vi "Get Ident.vi"(8 "Error In":errorcluster, 11 "reference in":refnum<class "Instrument.lvclass">) -> (0 "Error Out":errorcluster, 2 "Ident":string, 3 "reference out":refnum<class "Instrument.lvclass">)   [LabVIEW 2024, in "HAL.lvlib" / "Instrument.lvclass"]
uses:
  Instrument.lvclass
  Configurations/CFG Base/CFG Base.lvclass
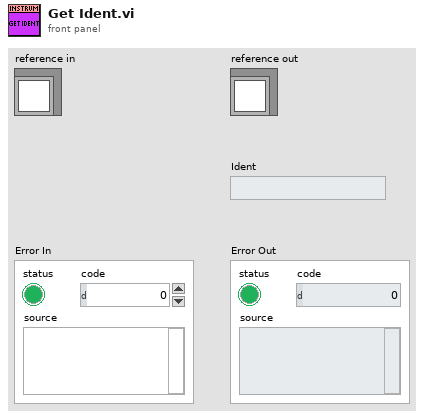
[diagram p1: front panel]
types:
  T1 = typedef "HAL.lvlib/Instrument.lvclass/ObjectAttributes.ctl" = cluster{"CFG Base":refnum<class "CFG Base.lvclass">, "Started Counter":i16}
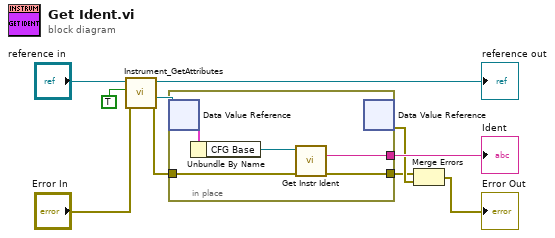
[diagram p0: block diagram]
diagram:
  n1 = call "Instrument_GetAttributes.vi"("Error In"="Error In", "OnlyGetDvrReference(False)"=TRUE, "reference in"="reference in") -> ("Error Out"=w2:errorcluster, "DataRef"=w3:refnum<data-value>, "reference out"=→"reference out":refnum<class "Instrument.lvclass">)  [unwired: 5 in, 1 out]
  n2 = in-place {
    in-place-border: [w13] -> w6
    in-place-border: w2 -> [w12]
    in-place-border: [w11] -> w1
    n3 = in-place-dvr #1(w3) -> (w14:T1)  [unwired: 1 out]
    n4 = Unbundle By Name(w14) -> ("CFG Base"=w15:refnum<class "CFG Base.lvclass">)
    n5 = call-dynamic "Get Instr Ident.vi"("error in"=w12, "CFG Base in"=w15) -> ("error out"=w11:errorcluster, "Instr Ident"=w13:string)  [unwired: 7 in, 1 out]
    n6 = in-place-dvr #1() -> (w5:errorcluster)  [unwired: 1 in, 1 out]
  }
  "Ident" <- w6
  n7 = Merge Errors(w1, w5) -> (→"Error Out":errorcluster)
